vi "_Check range I32.vi"(6 "Error Mode (Errors)":enum16{"Errors Off", "Errors", "Warnings"}(ring)=enum."Errors", 7 "Range Table Identifier":string, 8 "error in (no error)":errorcluster, 10 "I32 Value In":i32, 11 "VISA resource name":refnum<visa-resource-name>) -> (0 "error out":errorcluster, 2 "I32 Value Out":i32, 3 "VISA resource name out":refnum<visa-resource-name>)   [LabVIEW 2020, in "Rohde&Schwarz CMXP NR FR2 Measurement.lvlib"]
uses:
  <instrlib>/Rohde&Schwarz CMXP NR FR2 Measurement/Rohde&Schwarz CMXP NR FR2 Measurement.lvlib
  <instrlib>/Rohde&Schwarz CMXP NR FR2 Measurement/Private/rsidr_core.llb/type_Error_Codes.ctl
  <instrlib>/Rohde&Schwarz CMXP NR FR2 Measurement/Public/Utility/rsidr_core_global.vi
  <instrlib>/Rohde&Schwarz CMXP NR FR2 Measurement/Private/rsidr_core.llb/rsidr_core.lvlib
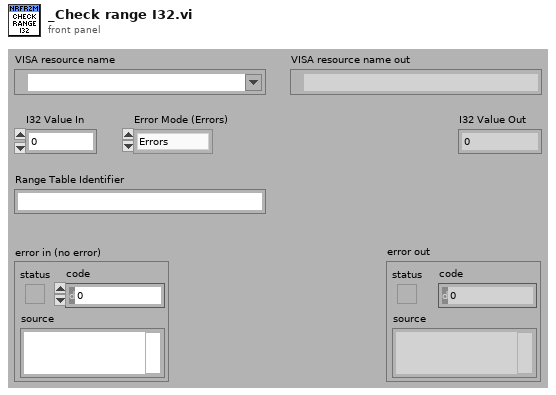
[diagram p1: front panel]
types:
  T1 = typedef "Rohde&Schwarz CMXP NR FR2 Measurement.lvlib/rsidr_core.lvlib/type_Error_Codes.ctl" = enum16{"No_error", "VISA_err_ResourceNotFound", "VISA_err_Timeout", "VISA_warn_MoreDataAvailable", "RS_err_MissingCallback", "RS_err_InvalidAttribute", "RS_err_InvalidValue", "RS_err_UnknownResource", "RS_err_AlreadyInitialized", "RS_err_InstrumentStatus", "RS_err_BadRepCapName", "RS_err_TypesMismatch", "RS_err_ValueNotSupported", "RS_err_InvalidRngTable", "RS_err_IDqueryFail", "RS_err_UnexpResponse", "VISA_warn_ConfigNotLoaded", "RS_err_AttributeNotReadable", "RS_err_AttributeNotWritable", "RS_err_InstrumentType", "RS_err_InstrumentOption", "VISA_err_InvalidSize", "RS_err_ReliabilityIndicator", "VISA_warn_UnknownStatus", "VISA_warn_TermCharRead", "VISA_err_IO_error", "RS_err_FunctionNotSupported", "VISA_warn_QueueEmpty"}
  T2 = cluster{"Name":string, "Type":enum16{"Range", "Coerced", "Discrete"}, "Entries":cluster{"Name":string, "Discrete or Min":dbl, "Max":dbl, "Coerced":dbl, "Command":string}[]}[]
  T3 = cluster{"Name":string, "Discrete or Min":dbl, "Max":dbl, "Coerced":dbl, "Command":string}[]
  T4 = cluster{"Name":string, "Discrete or Min":dbl, "Max":dbl, "Coerced":dbl, "Command":string}
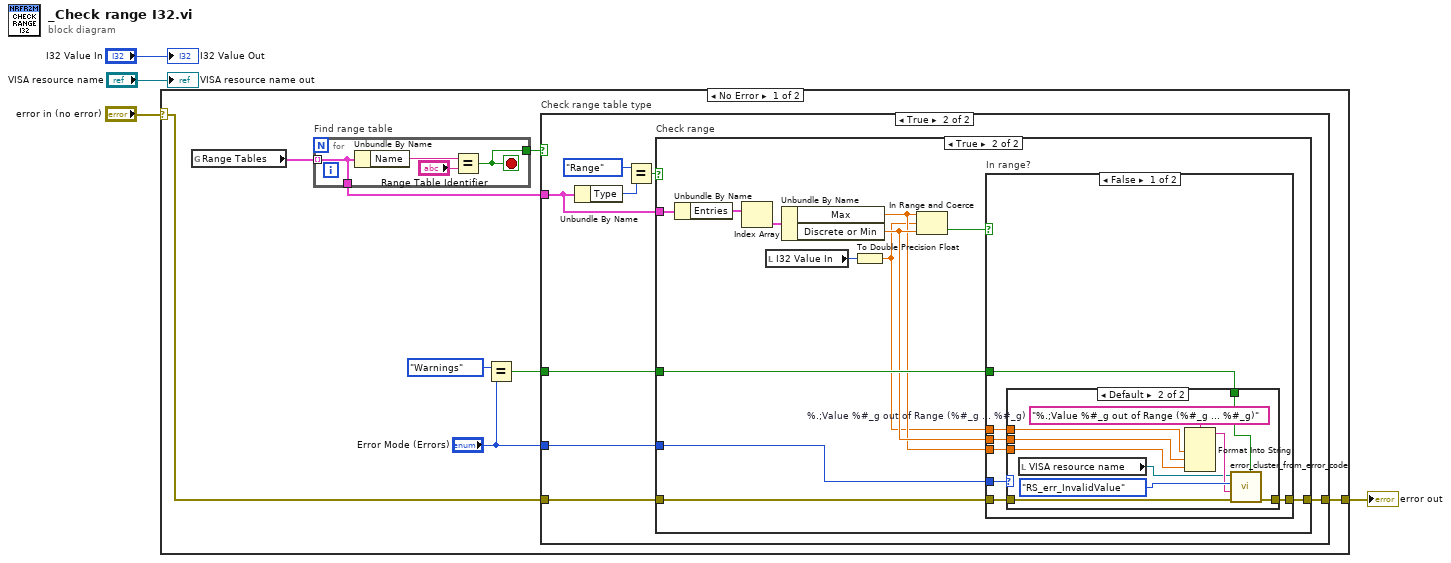
[diagram p0: block diagram]
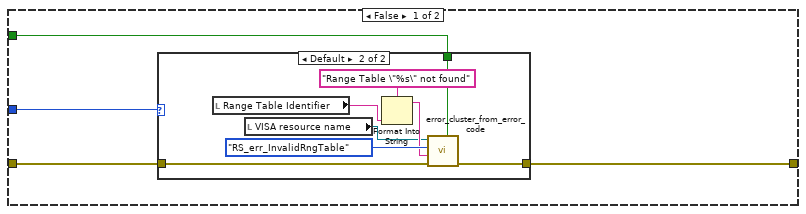
[diagram p2: hidden frame]
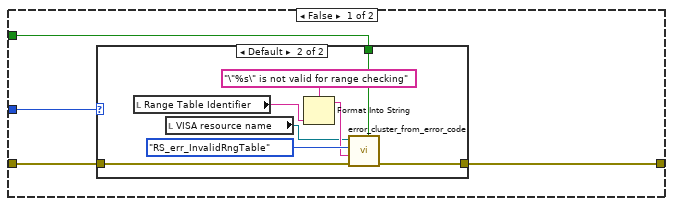
[diagram p4: hidden frame]
diagram:
  n1 = case shown="No Error" "error in (no error)" {
    selector: "error in (no error)" -> [w9 w82]
    tunnel: [w8 w82] -> w2
    frame No Error {
      n2 = global read "rsidr_core_global.vi" "Range Tables"() -> (w12:T2)
      n3 = for "Find range table" {
        tunnel: w12 -> [w79] mode=indexing
        tunnel: [w79] -> w11
        tunnel: [w78] -> w10
        stop <- w78 stop-if-true
        n4 = Unbundle By Name(w79) -> ("Name"=w80:string)
        n5 = Equal?(x=w80, y="Range Table Identifier") -> (x = y?=w78:bool)
      }
      n6 = Equal?(x=enum16{"Errors Off", "Errors", "Warnings"}."Warnings" ("Error Mode"), y="Error Mode (Errors)") -> (x = y?=w5:bool)
      n7 = case "Check range table type" shown="True" w10 {
        tunnel: w11 -> [_ w28]
        tunnel: w9 -> [w16 w31]
        tunnel: [w15 w30] -> w8
        tunnel: "Error Mode (Errors)" -> [w14 w27]
        tunnel: w5 -> [w13 w26]
        frame False {
          n8 = case shown="Default" w14 {
            tunnel: w16 -> [w17 w21]
            tunnel: [w17 w20] -> w15
            tunnel: w13 -> [_ w19]
            frame "Errors Off" {
            }
            frame Default {
              n9 = local read "Range Table Identifier"() -> (w25:string)
              n10 = local read "VISA resource name"() -> (w18:refnum<visa-resource-name>)
              n11 = Format Into String(format string="Range Table \"%s\" not found", w25) -> (resulting string=w22:string)  [unwired: 2 in, 1 out]
              n12 = call <instrlib>:"error_cluster_from_error_code.vi"("is warning? (False)"=w19, "error in"=w21, "error message (\"\")"=w22, "Error Enum in"=type_Error_Codes."RS_err_InvalidRngTable", "VISA resource name"=w18) -> ("error out"=w20:errorcluster)  [unwired: 5 in, 1 out]
            }
          }
        }
        frame True {
          n13 = Unbundle By Name(w28) -> ("Type"=w33:enum16{"Range", "Coerced", "Discrete"})
          n14 = Equal?(x=enum16{"Range", "Coerced", "Discrete"}."Range" ("Type"), y=w33) -> (x = y?=w29:bool)
          n15 = case "Check range" shown="True" w29 {
            tunnel: w31 -> [w37 w57]
            tunnel: [w36 w56] -> w30
            tunnel: w28 -> [_ w58]
            tunnel: w27 -> [w35 w55]
            tunnel: w26 -> [w34 w54]
            frame False {
              n16 = case shown="Default" w35 {
                tunnel: w37 -> [w38 w42]
                tunnel: [w38 w41] -> w36
                tunnel: w34 -> [_ w40]
                frame "Errors Off" {
                }
                frame Default {
                  n17 = local read "Range Table Identifier"() -> (w46:string)
                  n18 = local read "VISA resource name"() -> (w39:refnum<visa-resource-name>)
                  n19 = Format Into String(format string="\"%s\" is not valid for range checking", w46) -> (resulting string=w43:string)  [unwired: 2 in, 1 out]
                  n20 = call <instrlib>:"error_cluster_from_error_code.vi"("is warning? (False)"=w40, "error in"=w42, "error message (\"\")"=w43, "Error Enum in"=type_Error_Codes."RS_err_InvalidRngTable", "VISA resource name"=w39) -> ("error out"=w41:errorcluster)  [unwired: 5 in, 1 out]
                }
              }
            }
            frame True {
              n21 = Unbundle By Name(w58) -> ("Entries"=w53:T3)
              n22 = Index Array(array=w53) -> (element=w52:T4)  [unwired: 1 in]
              n23 = local read "I32 Value In"() -> (w50:i32)
              n24 = Unbundle By Name(w52) -> ("Max"=w48:dbl, "Discrete or Min"=w49:dbl)
              n25 = To Double Precision Float(number=w50) -> (double precision float=w47:dbl)
              n26 = In Range and Coerce(upper limit=w48, x=w47, lower limit=w49) -> (In Range?=w51:bool)  [unwired: 1 out]
              n27 = case "In range?" shown="False" w51 {
                tunnel: w57 -> [w65 w77]
                tunnel: [w64 w77] -> w56
                tunnel: w55 -> [w63 _]
                tunnel: w54 -> [w62 _]
                tunnel: w47 -> [w61 _]
                tunnel: w49 -> [w60 _]
                tunnel: w48 -> [w59 _]
                frame False {
                  n28 = case shown="Default" w63 {
                    tunnel: w65 -> [w66 w74]
                    tunnel: [w66 w73] -> w64
                    tunnel: w62 -> [_ w72]
                    tunnel: w61 -> [_ w69]
                    tunnel: w60 -> [_ w68]
                    tunnel: w59 -> [_ w67]
                    frame "Errors Off" {
                    }
                    frame Default {
                      w70 = "%.;Value %#_g out of Range (%#_g ... %#_g)"  # %.;Value %#_g out of Range (%#_g ... %#_g)
                      n29 = local read "VISA resource name"() -> (w71:refnum<visa-resource-name>)
                      n30 = Format Into String(format string=w70, w69, w68, w67) -> (resulting string=w75:string)  [unwired: 2 in, 1 out]
                      n31 = call <instrlib>:"error_cluster_from_error_code.vi"("is warning? (False)"=w72, "error in"=w74, "error message (\"\")"=w75, "Error Enum in"=type_Error_Codes."RS_err_InvalidValue", "VISA resource name"=w71) -> ("error out"=w73:errorcluster)  [unwired: 5 in, 1 out]
                    }
                  }
                }
                frame True {
                }
              }
            }
          }
        }
      }
    }
    frame Error {
    }
  }
  "error out" <- w2
  "VISA resource name out" <- "VISA resource name"
  "I32 Value Out" <- "I32 Value In"
